vi "Queue Demo.vi"() -> ()   [LabVIEW 2012]
uses:
  Queue.lvclass
panel:
  out "Items":variant[](array[variant])
  out "PeekItem":variant
  out "Items":variant[](array[variant])
  out "Item":variant
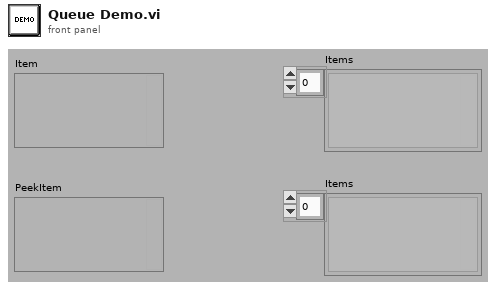
[diagram p1: front panel]
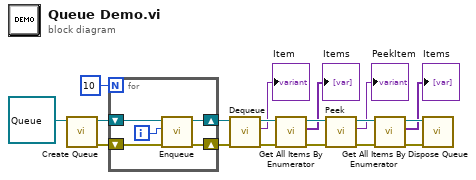
[diagram p0: block diagram]
diagram:
  n1 = call "Create Queue.vi"("Queue 输入"=refnum<class "Queue.lvclass"> refnum ("Queue.lvclass")) -> ("error out"=w16:errorcluster, "Queue 输出"=w17:refnum<class "Queue.lvclass">)  [unwired: 9 in]
  n2 = for {
    N: 10 -> [_]
    shift-right: [w20] -> w15
    shift-left: w17 -> [w23]
    shift-right: [w19] -> w14
    shift-left: w16 -> [w22]
    i -> [w21]
    n3 = call "Enqueue.vi"("error in (no error)"=w22, "Item"=w21, "Queue 输入"=w23) -> ("error out"=w19:errorcluster, "Queue 输出"=w20:refnum<class "Queue.lvclass">)  [unwired: 7 in]
  }
  n4 = call "Dequeue.vi"("error in (no error)"=w14, "Queue 输入"=w15) -> ("error out"=w12:errorcluster, "Item"=→"Item":variant, "Queue 输出"=w13:refnum<class "Queue.lvclass">)  [unwired: 7 in]
  n5 = call "Get All Items By Enumerator.vi"("error in (no error)"=w12, "Queue 输入"=w13) -> ("error out"=w10:errorcluster, "Items"=→"Items":variant[], "Queue 输出"=w11:refnum<class "Queue.lvclass">)  [unwired: 7 in]
  n6 = call "Peek.vi"("error in (no error)"=w10, "Queue 输入"=w11) -> ("error out"=w8:errorcluster, "Item"=→"PeekItem":variant, "Queue 输出"=w9:refnum<class "Queue.lvclass">)  [unwired: 7 in]
  n7 = call "Get All Items By Enumerator.vi"("error in (no error)"=w8, "Queue 输入"=w9) -> ("error out"=w6:errorcluster, "Items"=→"Items":variant[], "Queue 输出"=w7:refnum<class "Queue.lvclass">)  [unwired: 7 in]
  n8 = call "Dispose Queue.vi"("error in (no error)"=w6, "Queue 输入"=w7) -> ()  [unwired: 8 in, 2 out]
